vi "LED Driver.vi"(8 "State In":u8, 10 "LED Status":T1, 11 "Port":refnum<k21>) -> (0 "State Out":u8)   [LabVIEW 2014]
uses:
  Dash LED Status.ctl
  <vilib>/rvi/eio/common/nirviEmuTemplateMethod_errors.vi
  <vilib>/eio/EIONode/EIONode.xnode
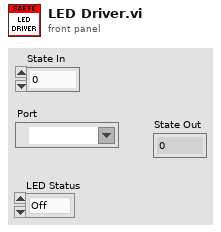
[diagram p1: front panel]
types:
  T1 = typedef "Dash LED Status.ctl" = enum16{"Off", "Flashing", "On"}
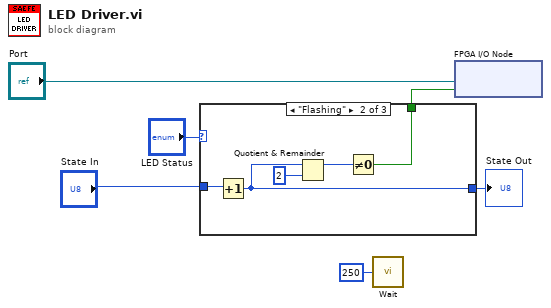
[diagram p0: block diagram]
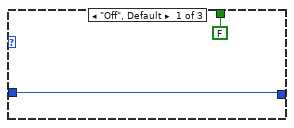
[diagram p2: hidden frame]
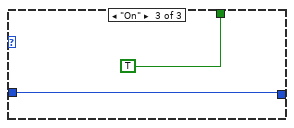
[diagram p3: hidden frame]
diagram:
  n1 = case shown="\"Flashing\"" "LED Status" {
    tunnel: [FALSE w9 TRUE] -> w5
    tunnel: "State In" -> [w7 w13 w14]
    tunnel: [w7 w12 w14] -> w2
    frame "Off", Default {
    }
    frame "Flashing" {
      n2 = Increment(x=w13) -> (x+1=w12:u8)
      n3 = Quotient & Remainder(x=w12, y=u8 2) -> (x-y*floor(x/y)=w10:u8)  [unwired: 1 out]
      n4 = Not Equal To 0?(x=w10) -> (x != 0?=w9:bool)
    }
    frame "On" {
    }
  }
  "State Out" <- w2
  n5 = call "Wait"("Count(mSec)"=u32 250) -> ()  [unwired: 1 out]
  n6 = xnode "FPGA I/O Node"("I/O Item"=w5, "FPGA I/O In"="Port") -> ()  [unwired: 1 out]
